vi "Do.vi"(8 "error in (no error)":errorcluster, 10 "Actor in":refnum<class "Actor.lvclass">, 11 "Change Laser Enable State":refnum<class "Change Laser Enable State.lvclass">) -> (0 "error out":errorcluster, 2 "Actor out":refnum<class "Actor.lvclass">)   [LabVIEW 2014, in "eCRDS Library.lvlib" / "Change Laser Enable State.lvclass"]
doc: "(<B>Filename</B>: Actor Framework.lvlib:Message.lvclass:Do.vi)\n\nDefines what a message does when it is received by an actor. Generally, a message instructs an actor to invoke one of its methods. By default, this method does nothing. A child class must override it to define behavior. Create a child class by using the Actor Framework Message Maker dialog box."
uses:
  Change Laser Enable State.lvclass
  <vilib>/ActorFramework/Actor/Actor.lvclass
  Change Laser Enable State.lvclass/Change Laser Enable State.ctl
  Instr Actor/Instr Actor.lvclass
  Controller/Messages/Update CVT/Update CVT Data.lvclass
  SuperActor/Ex Nested.lvclass/Ex Nested.ctl
  Controller/Messages/Update CVT/Update CVT Data.lvclass/Update CVT Data.ctl
  <vilib>/DAQmx/write.llb/DAQmx Write (Digital 1D Bool NChan 1Samp 1Line).vi
  <vilib>/DAQmx/write.llb/DAQmx Write (Digital Bool 1Line 1Point).vi
  Controller/Messages/Update CVT/Write Data.vi
  Controller/Messages/Update CVT/Write Group.vi
  Controller/Messages/Update CVT/Write tag.vi
  SuperActor/Read Log Session.vi
  <vilib>/DAQmx/miscellaneous.llb/DAQmx Fill In Error Info.vi
  <userlib>/_Session Fwk/Session - Root.lvclass
  reusable/Session APIs/Session Log/System Log.lvclass
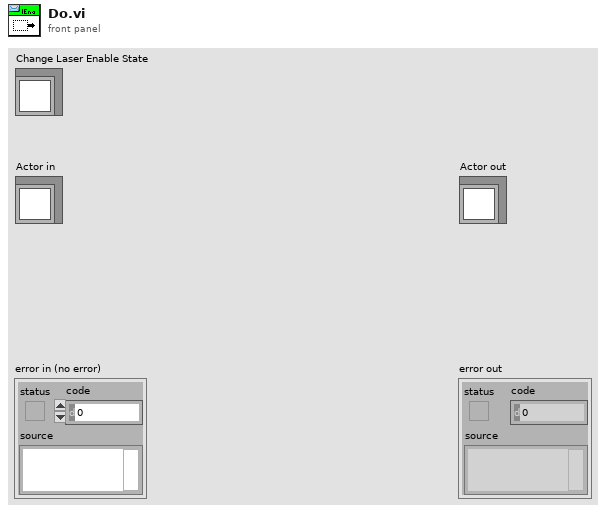
[diagram p1: front panel]
types:
  T1 = typedef "Session - Root.lvclass/Session Handle.ctl" = refnum<data-value>
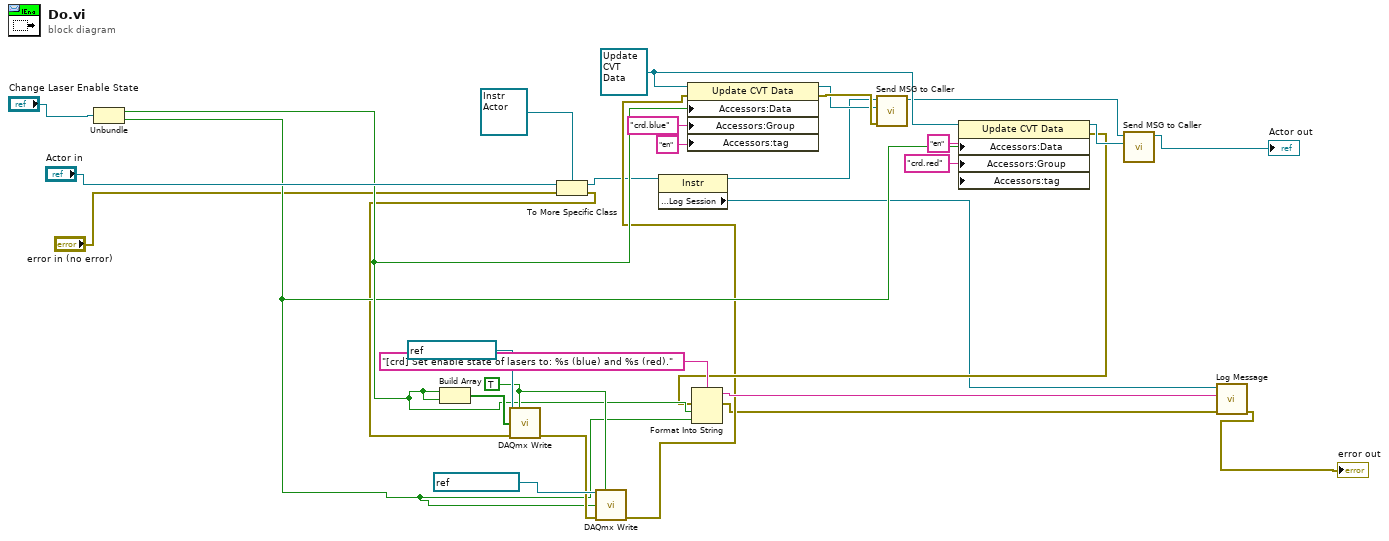
[diagram p0: block diagram]
diagram:
  w16 = refnum<class "Update CVT Data.lvclass"> refnum ("Controller.lvlib:Update CVT Data")
  w27 = TRUE ("auto start")
  n1 = Unbundle("Change Laser Enable State") -> (w19:bool, w15:bool)
  n2 = Build Array(w19, w19) -> (w30:bool[])
  n3 = To More Specific Class(target class=refnum<class "Instr Actor.lvclass"> refnum ("Instrument Lib:Instr"), reference="Actor in", error in="error in (no error)") -> (specific class reference=w3:refnum<class "Instr Actor.lvclass">, error out=w8:errorcluster)
  n4 = call-poly <vilib>:"DAQmx Write.vi"("task/channels in"=refnum<k21> "Blue Enable", "auto start"=w27, "data"=w30, "error in"=w8) -> ("error out"=w24:errorcluster)  [unwired: 9 in, 2 out]
  n5 = call-poly <vilib>:"DAQmx Write.vi"("task/channels in"=refnum<k21> "Red Enable", "auto start"=w27, "data"=w15, "error in"=w24) -> ("error out"=w5:errorcluster)  [unwired: 9 in, 2 out]
  n6 = property class="Instr"(reference=w3) -> (reference out=w1:refnum<class "Instr Actor.lvclass">, "Accessors:Log Session"=w2:T1)  [unwired: 1 in, 1 out]
  n7 = property class="Update CVT Data"(reference=w16, error in=w5, "Accessors:Data"=w19, "Accessors:Group"="crd.blue" ("Group"), "Accessors:tag"="en" ("tag")) -> (reference out=w17:refnum<class "Update CVT Data.lvclass">, error out=w18:errorcluster)
  n8 = call "Send MSG to Caller.vi"("error in"=w18, "Message"=w17, "Instr in"=w1) -> ("Instr out"=w11:refnum<class "Instr Actor.lvclass">)  [unwired: 7 in, 1 out]
  n9 = property class="Update CVT Data"(reference=w16, "Accessors:Data"=w15, "Accessors:Group"="crd.red" ("Group"), "Accessors:tag"="en" ("tag")) -> (reference out=w12:refnum<class "Update CVT Data.lvclass">, error out=w6:errorcluster)  [unwired: 1 in]
  n10 = Format Into String(format string="[crd] Set enable state of lasers to: %s (blue) and %s (red).", error in=w6, w19, w15) -> (resulting string=w25:string, error out=w4:errorcluster)  [unwired: 1 in]
  n11 = call "Send MSG to Caller.vi"("Message"=w12, "Instr in"=w11) -> ("Instr out"=→"Actor out":refnum<class "Instr Actor.lvclass">)  [unwired: 8 in, 1 out]
  n12 = call "Log Message.vi"("error in"=w4, "MSG In"=w25, "session in"=w2) -> ("error out"=→"error out":errorcluster)  [unwired: 7 in, 1 out]
